vi "Update Add Run Subpanel.vi"(8 "error in (no error)":errorcluster, 11 "Schedule Block in":refnum<class "Schedule Block.lvclass">) -> (0 "error out":errorcluster, 2 "Subpanel ref":refnum<vi>, 3 "Schedule Block out":refnum<class "Schedule Block.lvclass">)   [LabVIEW 2020, in "TALOS.lvlib" / "Run Utilities.lvlib" / "Schedule Block.lvclass"]
uses:
  Schedule Block.lvclass
  Schedule Block.lvclass/Schedule Block.ctl
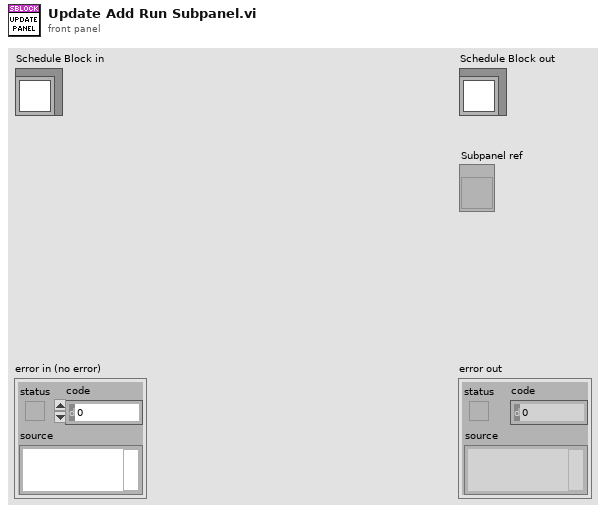
[diagram p1: front panel]
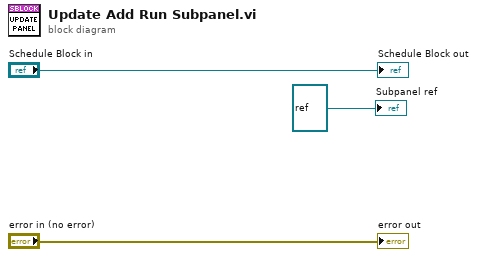
[diagram p0: block diagram]
diagram:
  "error out" <- "error in (no error)"
  "Schedule Block out" <- "Schedule Block in"
  "Subpanel ref" <- refnum<vi> refnum ("vi reference")
